vi "SplitTrame.vi"(0 "Données IN":string) -> (1 "Données OUT":string, 2 "Nouvelle commande":bool, 3 "Commande":string)   [LabVIEW 2011]
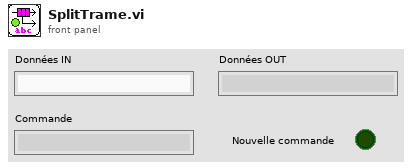
[diagram p1: front panel]
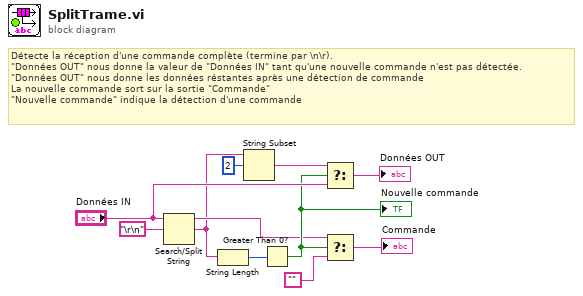
[diagram p0: block diagram]
diagram:
  # "Détecte la réception d'une commande complète (termine par \\n\\r).\n\"Données OUT\" nous donne la valeur de \"Données IN\" tant qu'une nouvelle commande n'est pas détectée.\n\"Données OUT\" nous donne les données réstantes après une détection de commande\nLa nouvelle commande sort sur la sortie \"Commande\"\n\"Nouvelle commande\" indique la détection d'une commande"
  n1 = Search/Split String(string="Données IN", search string/char (-)="\r\n") -> (substring before match=w8:string, match + rest of string=w5:string)  [unwired: 1 in, 1 out]
  n2 = String Length(string=w5) -> (length=w11:i32)
  n3 = String Subset(string=w5, offset (0)=2) -> (substring=w4:string)  [unwired: 1 in]
  n4 = Greater Than 0?(x=w11) -> (x > 0?=w9:bool)
  "Nouvelle commande" <- w9
  n5 = Select(t=w4, s=w9, f="Données IN") -> (s? t:f=→"Données OUT":string)
  n6 = Select(t=w8, s=w9, f="") -> (s? t:f=→"Commande":string)
